vi "Image Processing with Vision Assistant (FPGA).vi"() -> ()   [LabVIEW 2016]
uses:
  <vilib>/visionFPGA/Controls/IMAQ FPGA Image Size.ctl
  <vilib>/rvi/Emulation/niFpgaSctlEmulationGetInTimedLoop.vi
  <vilib>/rvi/Emulation/niFpgaProcessEmulError.vi
  <vilib>/rvi/Emulation/niFpgaGetClockAttributes.vi
  <vilib>/rvi/Emulation/niFpgaEmulationReportErrorSimple.vi
  <vilib>/visionFPGA/Basics/FIFO to Pixel Bus/IMAQ FPGA FIFO to Pixel Bus RGB32x1.vi
  <vilib>/rvi/DataTransferAndStorage/Container/Common/niFpgaContainerGetUniqueNameForEmu.vi
  <vilib>/rvi/DataTransferAndStorage/Container/Common/niFpgaContainerSetEmuInfo.vi
  <vilib>/rvi/eio/common/nirviEmuReportErrorAndStop.vi
  <vilib>/visionFPGA/Basics/Pixel Bus to FIFO/IMAQ FPGA Pixel Bus to FIFO U8x1.vi
  <vilib>/rvi/DataTransferAndStorage/Container/Common/niFpgaContainerExecOnDevCompGetState.vi
  <vilib>/rvi/Emulation/niFpgaEmulationIsFPGAContextNoSignature.vi
  <vilib>/rvi/errors/niFpgaSetErrorForExecOnDevCompSimple.vi
  <vilib>/rvi/FIFO/Fifo_Resource/nirvififoEmulationSetSize.vi
  <vilib>/rvi/FIFO/Fifo_Resource/nirviFifoEmulationQueueMgr.vi
  <instcachedir>/0/nirviFifoEmulationQueueMgr_E5CAEC123FF24DC58D834DCA3CDAA9B5.lvgen/nirviFifoEmulationQueueMgr_E5CAEC123FF24DC58D834DCA3CDAA9B5_008.vi
  <vilib>/rvi/FIFO/Fifo_Resource/nirvififoEmulationDetermineInputValidOut.vi
  <vilib>/rvi/FIFO/Fifo_Resource/nirvififoEmulationCreateLock.vi
  <vilib>/rvi/FIFO/Fifo_Resource/nirvififoEmulationObtainLock.vi
  <vilib>/rvi/FIFO/Fifo_Resource/nirvififoEmulationReleaseLock.vi
  <vilib>/rvi/occurrence/nirviWaitOnOccurrenceBase.vi
  <vilib>/rvi/errors/nirviReportUnexpectedCaseInternalError.vi
  <vilib>/rvi/errors/nirviReportUnexpectedCaseInternalError (U32).vi
  <vilib>/Utility/error.llb/Clear Errors.vi
  <vilib>/rvi/interface/RandomDataEmulation/niFpgaRandomDataHandleErrors.vi
  <vilib>/rvi/Emulation/niFpgaCriticalErrorInLSC.vi
  <vilib>/rvi/LocalResourceManager/LocalResourceManager.xnode
  <vilib>/rvi/DataTransferAndStorage/Container/XNode/niFpgaContainer.xnode
  <vilib>/rvi/FIFO/Fifo_Resource/niFpgaFifoEmulationRefIn.vi
  <vilib>/visionFPGA/NI_VDM_FPGA_Basics.lvlib
panel:
  out "ready to RecDOG2-3":bool=TRUE
  out "ready to RecDOG2-2":bool=TRUE
  out "ready to RecDOG2-1":bool=TRUE
  out "Ready For Input 4":bool=TRUE
  out "ready to RecDOG1-3":bool=TRUE
  out "Ready For Input 3":bool=TRUE
  out "ready to RecDOG1-2":bool=TRUE
  out "ready to RecDOG1-1":bool=TRUE
  out "ready to RecPic1 1":bool=TRUE
  out "Ready For Input 2":bool=TRUE
  out "Ready For Input":bool=TRUE
  out "Ready For Output":bool=TRUE
  out "EndOfImage":bool=TRUE
  out "Delay":i16=2
  in  "Image Size":T1={"Width"=640, "Height"=480}
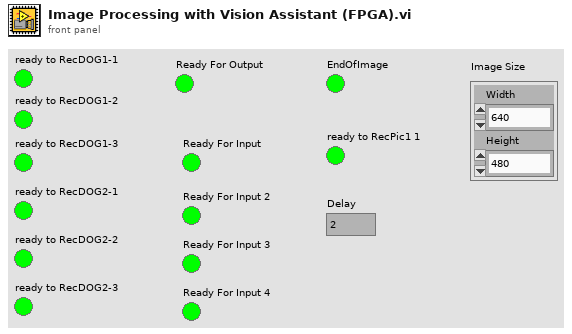
[diagram p1: front panel]
types:
  T1 = typedef "IMAQ FPGA Image Size.ctl" = cluster{"Width":u32, "Height":u32}
  T2 = typedef "IMAQ FPGA Pixel Bus RGB32x1.ctl" = cluster{"Pixel Data":cluster{"A":u8, "R/H":u8, "G/S":u8, "B/L":u8}, "DV":bool, "EOL":bool, "EOI":bool, "Data Type":enum16{"RGB32 x 1"}}
  T3 = typedef "IMAQ FPGA Pixel Bus u8x1.ctl" = cluster{"Pixel Data":u8, "DV":bool, "EOL":bool, "EOI":bool, "Data Type":enum16{"U8 x 1"}}
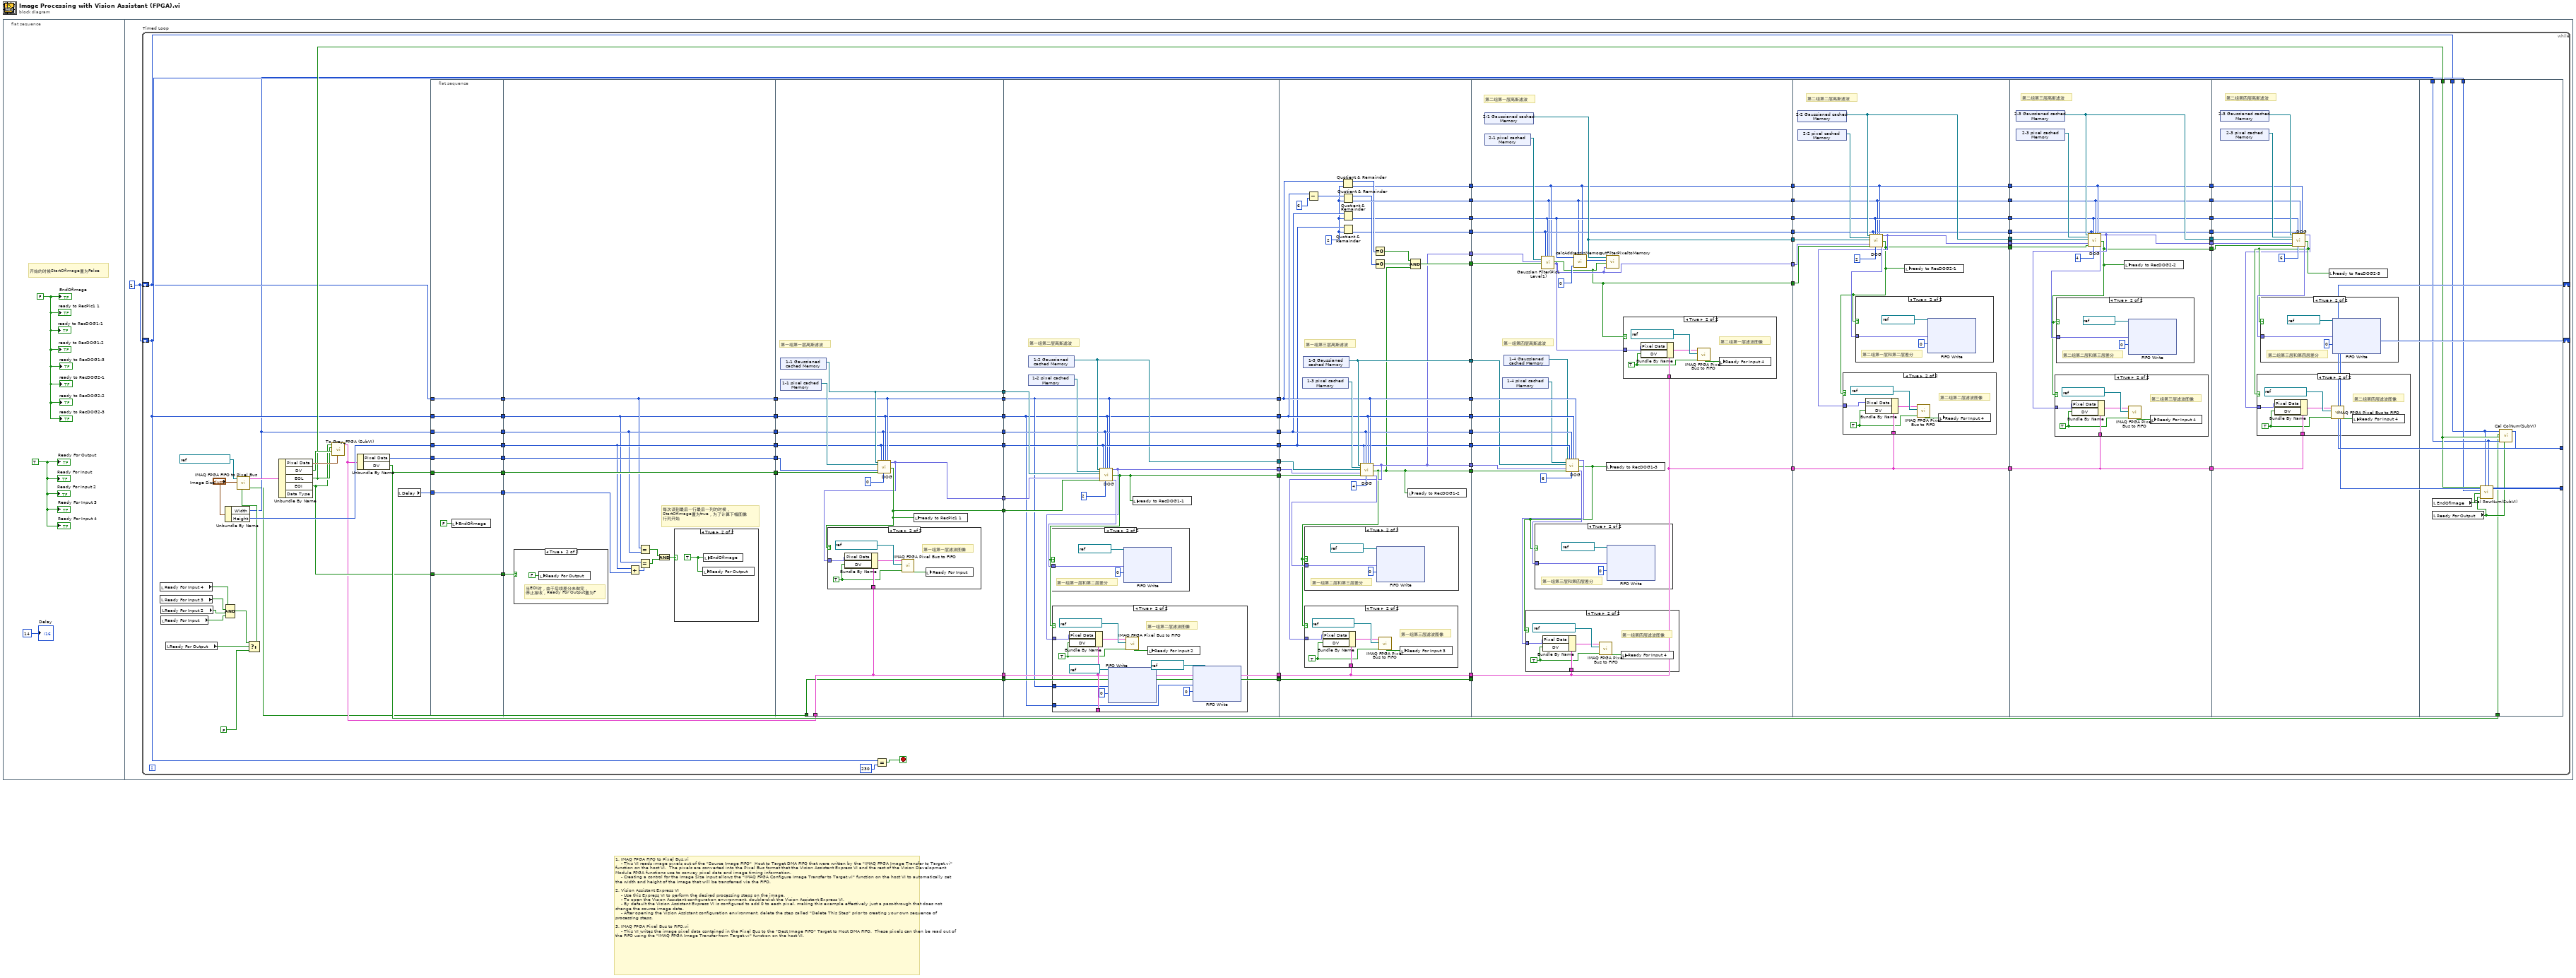
[diagram p0: block diagram]
diagram:
  # "1. IMAQ FPGA FIFO to Pixel Bus.vi\n    - This VI reads image pixels out of the \"Source Image FIFO\"  Host to Target DMA FIFO that were written by the \"IMAQ FPGA Image Transfer to Target.vi\" function on the host VI.  The pixels are converted into the Pixel Bus format that the Vision Assistant Express VI and the rest of the Vision Development Module FPGA functions use to convey pixel data and image timing information.\n    - Creating a control for the Image Size input allows the \"IMAQ FPGA Configure Image Transfer to Target.vi\" function on the host VI to automatically set the width and height of the image that will be transferred via the FIFO.\n\n2. Vision Assistant Express VI\n    - Use this Express VI to perform the desired processing steps on the image.\n    - To open the Vision Assistant configuration environment, double-click the Vision Assistant Express VI.\n    - By default the Vision Assistant Express VI is configured to add 0 to each pixel, making this example effectively just a pass-through that does not change the source image data.\n    - After opening the Vision Assistant configuration environment, delete the step called \"Delete This Step\" prior to creating your own sequence of processing steps.\n\n3. IMAQ FPGA Pixel Bus to FIFO.vi\n    - This VI writes the image pixel data contained in the Pixel Bus to the \"Dest Image FIFO\" Target to Host DMA FIFO.  These pixels can then be read out of the FIFO using the \"IMAQ FPGA Image Transfer from Target.vi\" function on the host VI."
  n1 = flat-sequence {
    frame #0 {
      w1 = FALSE
      w2 = TRUE ("Ready For Output")
      # "开始的时候StartOfImage置为False"
      "Delay" <- i16 14
      "EndOfImage" <- w1
      "Ready For Output" <- w2
      "Ready For Input" <- w2
      "Ready For Input 2" <- w2
      "ready to RecPic1 1" <- w1
      "ready to RecDOG1-1" <- w1
      "ready to RecDOG1-2" <- w1
      "Ready For Input 3" <- w2
      "ready to RecDOG1-3" <- w1
      "Ready For Input 4" <- w2
      "ready to RecDOG2-1" <- w1
      "ready to RecDOG2-2" <- w1
      "ready to RecDOG2-3" <- w1
    }
    frame #1 {
      w4 = i16 1 ("Output Line Count")
      n2 = while "Timed Loop" {
        shift-right: [w95] -> _
        shift-left: w4 -> [w87]
        shift-right: [w96] -> _
        shift-left: w4 -> [w86]
        stop <- w77 stop-if-true
        n3 = local read "Ready For Input 4"() -> (w59:bool)
        n4 = local read "Ready For Input 3"() -> (w62:bool)
        n5 = local read "Ready For Input 2"() -> (w63:bool)
        n6 = local read "Ready For Input"() -> (w56:bool)
        n7 = local read "Ready For Output"() -> (w90:bool)
        n8 = Unbundle By Name("Image Size") -> ("Width"=w78:u32, "Height"=w99:u32)
        n9 = Compound Arithmetic op=AND(w59, w62, w63, w56) -> (w66:bool)
        n10 = Select(t=w66, s=w90, f=FALSE) -> (s? t:f=w88:bool)
        n11 = call-poly <vilib>:"IMAQ FPGA FIFO to Pixel Bus.vi"("Ready For Output"=w88, "Image Size"="Image Size", "Source Image FIFO"=refnum<k21> "32it Source FIFO") -> ("Output Valid"=w67:bool, "Pixel Bus Out"=w102:T2)  [unwired: 6 in, 1 out]
        n12 = Unbundle By Name(w102) -> ("Pixel Data"=w100:cluster{"A":u8, "R/H":u8, "G/S":u8, "B/L":u8}, "DV"=w98:bool, "EOL"=w94:bool, "EOI"=w91:bool)  [unwired: 1 out]
        n13 = call "To Gray_FPGA (SubVI).vi"("Pixel Data"=w100, "DV"=w98, "EOL"=w94, "EOI"=w91) -> ("Pixel Bus In"=w68:T3)  [unwired: 7 in]
        n14 = Unbundle By Name(w68) -> ("Pixel Data"=w97:u8, "DV"=w93:bool)
        n15 = local read "Delay"() -> (w79:i16)
        n16 = flat-sequence {
          tunnel: w91 -> [w105]
          tunnel: w79 -> [w106]
          tunnel: w93 -> [w107]
          tunnel: w99 -> [w108]
          tunnel: w78 -> [w109]
          tunnel: w97 -> [w110]
          tunnel: w86 -> [w111]
          tunnel: w87 -> [w112]
          tunnel: [w112] -> w76
          tunnel: [w111] -> w75
          tunnel: [w110] -> w74
          tunnel: [w109] -> w73
          tunnel: [w108] -> w72
          tunnel: [w107] -> w71
          tunnel: [w106] -> w70
          tunnel: [w105] -> w69
          tunnel: [w118] -> w85
          tunnel: [w117] -> w84
          tunnel: [w116] -> w83
          tunnel: [w115] -> w82
          tunnel: [w114] -> w81
          tunnel: [w113] -> w80
          tunnel: w76 -> [w113]
          tunnel: w75 -> [w114]
          tunnel: w74 -> [w117]
          tunnel: w73 -> [w115]
          tunnel: w72 -> [w116]
          tunnel: w71 -> [w118]
          tunnel: w70 -> [w120]
          tunnel: w69 -> [w121]
          tunnel: w85 -> [w136]
          tunnel: w84 -> [w137]
          tunnel: w83 -> [w128]
          tunnel: w82 -> [w129]
          tunnel: w81 -> [w131]
          tunnel: w80 -> [w130]
          tunnel: w68 -> [w139]
          tunnel: w67 -> [w138]
          tunnel: [w139] -> w65
          tunnel: [w138] -> w64
          tunnel: [w131] -> w55
          tunnel: [w130] -> w54
          tunnel: [w129] -> w53
          tunnel: [w128] -> w52
          tunnel: [w134] -> w51
          tunnel: [w135] -> w50
          tunnel: [w132] -> w47
          tunnel: w65 -> [w149]
          tunnel: w64 -> [w148]
          tunnel: [w148] -> w61
          tunnel: [w149] -> w60
          tunnel: w55 -> [w147]
          tunnel: w54 -> [w146]
          tunnel: w53 -> [w155]
          tunnel: w52 -> [w154]
          tunnel: w51 -> [w157]
          tunnel: w50 -> [w156]
          tunnel: [w150] -> w49
          tunnel: [w151] -> w48
          tunnel: w47 -> [w158]
          tunnel: [w147] -> w46
          tunnel: [w146] -> w45
          tunnel: [w155] -> w44
          tunnel: [w154] -> w43
          tunnel: [w153] -> w35
          tunnel: w61 -> [w176]
          tunnel: w60 -> [w177]
          tunnel: [w176] -> w58
          tunnel: [w177] -> w57
          tunnel: w49 -> [w202]
          tunnel: w48 -> [w201]
          tunnel: w46 -> [w193]
          tunnel: w45 -> [w195]
          tunnel: w44 -> [w184]
          tunnel: w43 -> [w182]
          tunnel: [w179] -> w42
          tunnel: [w178] -> w41
          tunnel: [w193] -> w40
          tunnel: [w195] -> w39
          tunnel: [w184] -> w38
          tunnel: [w182] -> w37
          tunnel: [w198] -> w36
          tunnel: w35 -> [w197]
          tunnel: [w183] -> w34
          tunnel: [w180] -> w33
          tunnel: [w194] -> w32
          tunnel: [w190] -> w31
          tunnel: [w179] -> w30
          tunnel: [w187] -> w29
          tunnel: w58 -> [_]
          tunnel: w57 -> [w213]
          tunnel: w42 -> [w237]
          tunnel: w41 -> [w236]
          tunnel: w40 -> [w235]
          tunnel: w39 -> [w234]
          tunnel: w38 -> [w233]
          tunnel: w37 -> [w232]
          tunnel: w36 -> [w229]
          tunnel: w34 -> [w220]
          tunnel: w33 -> [w221]
          tunnel: w32 -> [w217]
          tunnel: w31 -> [w219]
          tunnel: w30 -> [w225]
          tunnel: w29 -> [w218]
          tunnel: [w222] -> w28
          tunnel: [w214] -> w27
          tunnel: [w212] -> w26
          tunnel: [w221] -> w25
          tunnel: [w220] -> w24
          tunnel: [w217] -> w23
          tunnel: [w219] -> w22
          tunnel: [w213] -> w7
          tunnel: w28 -> [w264]
          tunnel: w27 -> [w263]
          tunnel: w26 -> [w262]
          tunnel: w25 -> [w259]
          tunnel: w24 -> [w260]
          tunnel: w23 -> [w258]
          tunnel: w22 -> [w257]
          tunnel: [w261] -> w21
          tunnel: [w257] -> w20
          tunnel: [w258] -> w19
          tunnel: [w260] -> w18
          tunnel: [w259] -> w17
          tunnel: [w255] -> w16
          tunnel: [w253] -> w15
          tunnel: w7 -> [w254]
          tunnel: [w254] -> w6
          tunnel: w21 -> [w287]
          tunnel: w20 -> [w283]
          tunnel: w19 -> [w282]
          tunnel: w18 -> [w281]
          tunnel: w17 -> [w280]
          tunnel: w16 -> [w286]
          tunnel: w15 -> [w285]
          tunnel: [w278] -> w14
          tunnel: [w277] -> w13
          tunnel: [w284] -> w12
          tunnel: [w283] -> w11
          tunnel: [w282] -> w10
          tunnel: [w281] -> w9
          tunnel: [w280] -> w8
          tunnel: w6 -> [w276]
          tunnel: [w276] -> w5
          tunnel: w14 -> [w309]
          tunnel: w13 -> [w308]
          tunnel: w12 -> [w307]
          tunnel: w11 -> [w306]
          tunnel: w10 -> [w305]
          tunnel: w9 -> [w304]
          tunnel: w8 -> [w303]
          tunnel: w5 -> [w299]
          tunnel: w86 -> [w322]
          tunnel: w93 -> [w323]
          tunnel: w94 -> [w328]
          tunnel: w87 -> [w324]
          tunnel: w78 -> [w327]
          tunnel: [w330] -> w96
          tunnel: [w329] -> w95
          frame #0 {
            n17 = local write "EndOfImage"(FALSE ("StartOfImage")) -> ()
          }
          frame #1 {
            # "每次读到最后一行最后一列的时候，\nStartOfImage置为true，为了计算下幅图像\n行列开始"
            n18 = case shown="True" w121 {
              frame False {
              }
              frame True {
                # "当EOI时，由于后续差分未做完，\n停止接收，Ready For Output置为F"
                n19 = local write "Ready For Output"(FALSE ("Ready For Output")) -> ()
              }
            }
            n20 = Add(x=w116, y=w120) -> (x+y=w119:u32)
            n21 = Equal?(x=w114, y=w115) -> (x = y?=w123:bool)
            n22 = Equal?(x=w113, y=w119) -> (x = y?=w124:bool)
            n23 = And(x=w123, y=w124) -> (x .and. y?=w122:bool)
            n24 = case shown="True" w122 {
              frame False {
              }
              frame True {
                w125 = TRUE ("StartOfImage")
                n25 = local write "Ready For Output"(w125) -> ()
                n26 = local write "EndOfImage"(w125) -> ()
              }
            }
          }
          frame #2 {
            # "第一组第一层高斯滤波"
            n27 = xnode "1-1 Gaussianed cached Memory"() -> ("Memory Out"=w132:refnum<k21>)
            n28 = xnode "1-1 pixel cached Memory"() -> ("Memory Out"=w133:refnum<k21>)
            n29 = call "DOG.vi"("Gaussianed cached Memory"=w132, "pixel cached Memory"=w133, "Data in"=w137, "DV in"=w136, "Height"=w128, "Width"=w129, "DelayRowCount"=i16 0, "Rows"=w130, "Cols"=w131) -> ("GaussianFilterData out"=w134:fxp<+,12,12>, "DV out"=w135:bool)  [unwired: 8 in, 1 out]
            n30 = case shown="True" w135 {
              tunnel: w134 -> [_ w141]
              tunnel: w139 -> [_ w142]
              frame False {
              }
              frame True {
                w140 = TRUE ("Input Valid")
                # "第一组第一层滤波图像"
                n31 = Bundle By Name(cluster=w142, "Pixel Data"=w141, "DV"=w140) -> (w143:T3)
                n32 = call-poly <vilib>:"IMAQ FPGA Pixel Bus to FIFO.vi"("Input Valid"=w140, "Destination Image FIFO"=refnum<k21> "Gaussian 1-1", "Pixel Bus In"=w143) -> ("Ready for Input"=w144:bool)  [unwired: 8 in]
                n33 = local write "Ready For Input"(w144) -> ()
              }
            }
            n34 = local write "ready to RecPic1 1"(w135) -> ()
          }
          frame #3 {
            # "第一组第二层高斯滤波"
            n35 = xnode "1-2 Gaussianed cached Memory"() -> ("Memory Out"=w153:refnum<k21>)
            n36 = xnode "1-2 pixel cached Memory"() -> ("Memory Out"=w159:refnum<k21>)
            n37 = call "DOG.vi"("Gaussianed cached Memory"=w153, "pixel cached Memory"=w159, "preGaussianed cached Memory"=w158, "Data in"=w157, "DV in"=w156, "Height"=w154, "Width"=w155, "DelayRowCount"=i16 2, "Rows"=w146, "Cols"=w147) -> ("GaussianFilterData out"=w151:fxp<+,12,12>, "DV out"=w150:bool, "DOG Out"=w152:fxp<+/-,13,13>)  [unwired: 7 in]
            n38 = case shown="True" w150 {
              tunnel: w152 -> [_ w173]
              frame False {
              }
              frame True {
                # "第一组第一层和第二层差分"
                n39 = xnode ("FIFO Write")("Element"=w173, "Timeout"=0, "FIFO In"=refnum<k21> "DOG 1-1") -> ()  [unwired: 2 out]
              }
            }
            n40 = case shown="True" w150 {
              tunnel: w151 -> [_ w168]
              tunnel: w149 -> [_ w169]
              tunnel: w147 -> [_ w165]
              tunnel: w146 -> [_ w163]
              frame False {
              }
              frame True {
                w167 = TRUE ("Input Valid")
                # "第一组第二层滤波图像"
                n41 = Bundle By Name(cluster=w169, "Pixel Data"=w168, "DV"=w167) -> (w170:T3)
                n42 = xnode ("FIFO Write")("Element"=w165, "Timeout"=0, "FIFO In"=refnum<k21> "testCols") -> ()  [unwired: 2 out]
                n43 = call-poly <vilib>:"IMAQ FPGA Pixel Bus to FIFO.vi"("Input Valid"=w167, "Destination Image FIFO"=refnum<k21> "Gaussian 1-2", "Pixel Bus In"=w170) -> ("Ready for Input"=w171:bool)  [unwired: 8 in]
                n44 = local write "Ready For Input 2"(w171) -> ()
                n45 = xnode ("FIFO Write")("Element"=w163, "Timeout"=0, "FIFO In"=refnum<k21> "testRows") -> ()  [unwired: 2 out]
              }
            }
            n46 = local write "ready to RecDOG1-1"(w150) -> ()
          }
          frame #4 {
            w181 = u32 2 ("y")
            # "第一组第三层高斯滤波"
            n47 = xnode "1-3 pixel cached Memory"() -> ("Memory Out"=w200:refnum<k21>)
            n48 = xnode "1-3 Gaussianed cached Memory"() -> ("Memory Out"=w198:refnum<k21>)
            n49 = Subtract(x=w195, y=i16 6) -> (x-y=w186:i16)
            n50 = Quotient & Remainder(x=w193, y=w181) -> (x-y*floor(x/y)=w192:u32, floor(x/y)=w190:u32)
            n51 = Quotient & Remainder(x=w186, y=w181) -> (x-y*floor(x/y)=w191:u32, floor(x/y)=w194:u32)
            n52 = Quotient & Remainder(x=w184, y=w181) -> (floor(x/y)=w183:u32)  [unwired: 1 out]
            n53 = Quotient & Remainder(x=w182, y=w181) -> (floor(x/y)=w180:u32)  [unwired: 1 out]
            n54 = call "DOG.vi"("Gaussianed cached Memory"=w198, "pixel cached Memory"=w200, "preGaussianed cached Memory"=w197, "Data in"=w201, "DV in"=w202, "Height"=w182, "Width"=w184, "DelayRowCount"=i16 4, "Rows"=w195, "Cols"=w193) -> ("GaussianFilterData out"=w179:fxp<+,12,12>, "DV out"=w178:bool, "DOG Out"=w199:fxp<+/-,13,13>)  [unwired: 7 in]
            n55 = case shown="True" w178 {
              tunnel: w199 -> [_ w210]
              frame False {
              }
              frame True {
                # "第一组第二层和第三层差分"
                n56 = xnode ("FIFO Write")("Element"=w210, "Timeout"=0, "FIFO In"=refnum<k21> "DOG 1-2") -> ()  [unwired: 2 out]
              }
            }
            n57 = case shown="True" w178 {
              tunnel: w179 -> [_ w204]
              tunnel: w177 -> [_ w205]
              frame False {
              }
              frame True {
                w203 = TRUE ("Input Valid")
                # "第一组第三层滤波图像"
                n58 = Bundle By Name(cluster=w205, "Pixel Data"=w204, "DV"=w203) -> (w206:T3)
                n59 = call-poly <vilib>:"IMAQ FPGA Pixel Bus to FIFO.vi"("Input Valid"=w203, "Destination Image FIFO"=refnum<k21> "Gaussian 1-3", "Pixel Bus In"=w206) -> ("Ready for Input"=w207:bool)  [unwired: 8 in]
                n60 = local write "Ready For Input 3"(w207) -> ()
              }
            }
            n61 = Equal To 0?(x=w192) -> (x = 0?=w189:bool)
            n62 = Equal To 0?(x=w191) -> (x = 0?=w188:bool)
            n63 = local write "ready to RecDOG1-2"(w178) -> ()
            n64 = Compound Arithmetic op=AND(w189, w188, w178) -> (w187:bool)
          }
          frame #5 {
            # "第二组第一层高斯滤波"
            # "第一组第四层高斯滤波"
            n65 = xnode "2-1 Gaussianed cached Memory"() -> ("Memory Out"=w222:refnum<k21>)
            n66 = xnode "2-1 pixel cached Memory"() -> ("Memory Out"=w226:refnum<k21>)
            n67 = xnode "1-4 pixel cached Memory"() -> ("Memory Out"=w230:refnum<k21>)
            n68 = xnode "1-4 Gaussianed cached Memory"() -> ("Memory Out"=w231:refnum<k21>)
            n69 = call "Gaussian Filter(Pic1 Level1).vi"("Memory In"=w226, "Data In"=w225, "DV In"=w218, "Height"=w221, "Width"=w220, "Rows"=w217, "Cols"=w219) -> ("DV out"=w212:bool, "Data Out"=w214:fxp<+,12,12>)  [unwired: 11 in]
            n70 = call "DOG.vi"("Gaussianed cached Memory"=w231, "pixel cached Memory"=w230, "preGaussianed cached Memory"=w229, "Data in"=w237, "DV in"=w236, "Height"=w232, "Width"=w233, "DelayRowCount"=i16 6, "Rows"=w234, "Cols"=w235) -> ("GaussianFilterData out"=w216:fxp<+,12,12>, "DV out"=w215:bool, "DOG Out"=w228:fxp<+/-,13,13>)  [unwired: 7 in]
            n71 = case shown="True" w215 {
              tunnel: w216 -> [_ w245]
              tunnel: w213 -> [_ w246]
              frame False {
              }
              frame True {
                w244 = TRUE ("Input Valid")
                # "第一组第四层滤波图像"
                n72 = Bundle By Name(cluster=w246, "Pixel Data"=w245, "DV"=w244) -> (w247:T3)
                n73 = call-poly <vilib>:"IMAQ FPGA Pixel Bus to FIFO.vi"("Input Valid"=w244, "Destination Image FIFO"=refnum<k21> "Gaussian 1-4", "Pixel Bus In"=w247) -> ("Ready for Input"=w248:bool)  [unwired: 8 in]
                n74 = local write "Ready For Input 4"(w248) -> ()
              }
            }
            n75 = case shown="True" w215 {
              tunnel: w228 -> [_ w251]
              frame False {
              }
              frame True {
                # "第一组第三层和第四层差分"
                n76 = xnode ("FIFO Write")("Element"=w251, "Timeout"=0, "FIFO In"=refnum<k21> "DOG 1-3") -> ()  [unwired: 2 out]
              }
            }
            n77 = call "calcAddressInMemory.vi"("Width"=w220, "Rows"=w217, "delayRowCount"=i16 0, "Cols"=w219) -> ("addressInMemory"=w223:u32)  [unwired: 5 in]
            n78 = local write "ready to RecDOG1-3"(w215) -> ()
            n79 = call "putFilterPixeltoMemory.vi"("Data In"=w214, "DV in"=w212, "addressInMemory"=w223, "Memory in"=w222) -> ()
            n80 = case shown="True" w212 {
              tunnel: w214 -> [_ w239]
              tunnel: w213 -> [_ w240]
              frame False {
              }
              frame True {
                w238 = TRUE ("Input Valid")
                # "第二组第一层滤波图像"
                n81 = Bundle By Name(cluster=w240, "Pixel Data"=w239, "DV"=w238) -> (w241:T3)
                n82 = call-poly <vilib>:"IMAQ FPGA Pixel Bus to FIFO.vi"("Input Valid"=w238, "Destination Image FIFO"=refnum<k21> "Gaussian 2-1", "Pixel Bus In"=w241) -> ("Ready for Input"=w242:bool)  [unwired: 8 in]
                n83 = local write "Ready For Input 4"(w242) -> ()
              }
            }
          }
          frame #6 {
            # "第二组第二层高斯滤波"
            n84 = xnode "2-2 Gaussianed cached Memory"() -> ("Memory Out"=w261:refnum<k21>)
            n85 = xnode "2-2 pixel cached Memory"() -> ("Memory Out"=w265:refnum<k21>)
            n86 = call "DOG.vi"("Gaussianed cached Memory"=w261, "pixel cached Memory"=w265, "preGaussianed cached Memory"=w264, "Data in"=w263, "DV in"=w262, "Height"=w259, "Width"=w260, "DelayRowCount"=i16 2, "Rows"=w258, "Cols"=w257) -> ("GaussianFilterData out"=w255:fxp<+,12,12>, "DV out"=w253:bool, "DOG Out"=w256:fxp<+/-,13,13>)  [unwired: 7 in]
            n87 = case shown="True" w253 {
              tunnel: w255 -> [_ w268]
              tunnel: w254 -> [_ w269]
              frame False {
              }
              frame True {
                w267 = TRUE ("Input Valid")
                # "第二组第二层滤波图像"
                n88 = Bundle By Name(cluster=w269, "Pixel Data"=w268, "DV"=w267) -> (w270:T3)
                n89 = call-poly <vilib>:"IMAQ FPGA Pixel Bus to FIFO.vi"("Input Valid"=w267, "Destination Image FIFO"=refnum<k21> "Gaussian 1-4", "Pixel Bus In"=w270) -> ("Ready for Input"=w271:bool)  [unwired: 8 in]
                n90 = local write "Ready For Input 4"(w271) -> ()
              }
            }
            n91 = case shown="True" w253 {
              tunnel: w256 -> [_ w274]
              frame False {
              }
              frame True {
                # "第二组第一层和第二层差分"
                n92 = xnode ("FIFO Write")("Element"=w274, "Timeout"=0, "FIFO In"=refnum<k21> "DOG 2-1") -> ()  [unwired: 2 out]
              }
            }
            n93 = local write "ready to RecDOG2-1"(w253) -> ()
          }
          frame #7 {
            # "第二组第三层高斯滤波"
            n94 = xnode "2-3 Gaussianed cached Memory"() -> ("Memory Out"=w284:refnum<k21>)
            n95 = xnode "2-3 pixel cached Memory"() -> ("Memory Out"=w288:refnum<k21>)
            n96 = call "DOG.vi"("Gaussianed cached Memory"=w284, "pixel cached Memory"=w288, "preGaussianed cached Memory"=w287, "Data in"=w286, "DV in"=w285, "Height"=w280, "Width"=w281, "DelayRowCount"=i16 4, "Rows"=w282, "Cols"=w283) -> ("GaussianFilterData out"=w278:fxp<+,12,12>, "DV out"=w277:bool, "DOG Out"=w279:fxp<+/-,13,13>)  [unwired: 7 in]
            n97 = case shown="True" w277 {
              tunnel: w278 -> [_ w291]
              tunnel: w276 -> [_ w292]
              frame False {
              }
              frame True {
                w290 = TRUE ("Input Valid")
                # "第二组第三层滤波图像"
                n98 = Bundle By Name(cluster=w292, "Pixel Data"=w291, "DV"=w290) -> (w293:T3)
                n99 = call-poly <vilib>:"IMAQ FPGA Pixel Bus to FIFO.vi"("Input Valid"=w290, "Destination Image FIFO"=refnum<k21> "Gaussian 1-4", "Pixel Bus In"=w293) -> ("Ready for Input"=w294:bool)  [unwired: 8 in]
                n100 = local write "Ready For Input 4"(w294) -> ()
              }
            }
            n101 = case shown="True" w277 {
              tunnel: w279 -> [_ w297]
              frame False {
              }
              frame True {
                # "第二组第二层和第三层差分"
                n102 = xnode ("FIFO Write")("Element"=w297, "Timeout"=0, "FIFO In"=refnum<k21> "DOG 2-2") -> ()  [unwired: 2 out]
              }
            }
            n103 = local write "ready to RecDOG2-2"(w277) -> ()
          }
          frame #8 {
            # "第二组第四层高斯滤波"
            n104 = xnode "2-3 Gaussianed cached Memory"() -> ("Memory Out"=w310:refnum<k21>)
            n105 = xnode "2-3 pixel cached Memory"() -> ("Memory Out"=w311:refnum<k21>)
            n106 = call "DOG.vi"("Gaussianed cached Memory"=w310, "pixel cached Memory"=w311, "preGaussianed cached Memory"=w307, "Data in"=w309, "DV in"=w308, "Height"=w303, "Width"=w304, "DelayRowCount"=i16 6, "Rows"=w305, "Cols"=w306) -> ("GaussianFilterData out"=w300:fxp<+,12,12>, "DV out"=w301:bool, "DOG Out"=w302:fxp<+/-,13,13>)  [unwired: 7 in]
            n107 = case shown="True" w301 {
              tunnel: w300 -> [_ w314]
              tunnel: w299 -> [_ w315]
              frame False {
              }
              frame True {
                w313 = TRUE ("Input Valid")
                # "第二组第四层滤波图像"
                n108 = Bundle By Name(cluster=w315, "Pixel Data"=w314, "DV"=w313) -> (w316:T3)
                n109 = call-poly <vilib>:"IMAQ FPGA Pixel Bus to FIFO.vi"("Input Valid"=w313, "Destination Image FIFO"=refnum<k21> "Gaussian 1-4", "Pixel Bus In"=w316) -> ("Ready for Input"=w317:bool)  [unwired: 8 in]
                n110 = local write "Ready For Input 4"(w317) -> ()
              }
            }
            n111 = case shown="True" w301 {
              tunnel: w302 -> [_ w320]
              frame False {
              }
              frame True {
                # "第二组第三层和第四层差分"
                n112 = xnode ("FIFO Write")("Element"=w320, "Timeout"=0, "FIFO In"=refnum<k21> "DOG 2-3") -> ()  [unwired: 2 out]
              }
            }
            n113 = local write "ready to RecDOG2-3"(w301) -> ()
          }
          frame #9 {
            n114 = local read "EndOfImage"() -> (w325:bool)
            n115 = local read "Ready For Output"() -> (w326:bool)
            n116 = call "Cal RowNum(SubVI).vi"("Width"=w327, "curCol"=w322, "Ready For Input"=w326, "EndOfImage"=w325, "curRow"=w324, "EOL"=w328) -> ("nextRow"=w329:i16)  [unwired: 5 in]
            n117 = call "Cal ColNum(SubVI).vi"("Ready For Input"=w326, "Width"=w327, "EOL"=w328, "DV"=w323, "curColNum"=w322) -> ("nextColNum"=w330:i16)  [unwired: 6 in]
          }
        }
        n118 = Equal?(x=w87, y=i16 230) -> (x = y?=w77:bool)
      }
    }
  }
